vi "virtualOSA_model_code.vi"(11 "virtual OSA model":T1) -> (1 "OSA series":enum16{"OSA200", "OSA300", "UNKNOWN"}(ring), 3 "virtualOSA code":u16)   [LabVIEW 2010, in "OSA.lvclass"]
uses:
  OSA.lvclass
  _misc/Thorlabs_FTS_misc.llb/OSA_virtualModel.ctl
  OSA20X_misc.lvlib
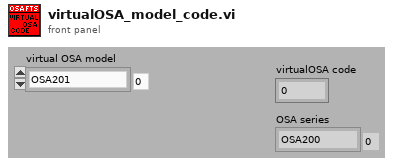
[diagram p1: front panel]
types:
  T1 = typedef "OSA20X_misc.lvlib/OSA_virtualModel.ctl" = enum16{"OSA201", "OSA201C", "OSA202", "OSA202C", "OSA203", "OSA203B", "OSA203C", "OSA205", "OSA205C", "REDSTONE301", "REDSTONE305"}
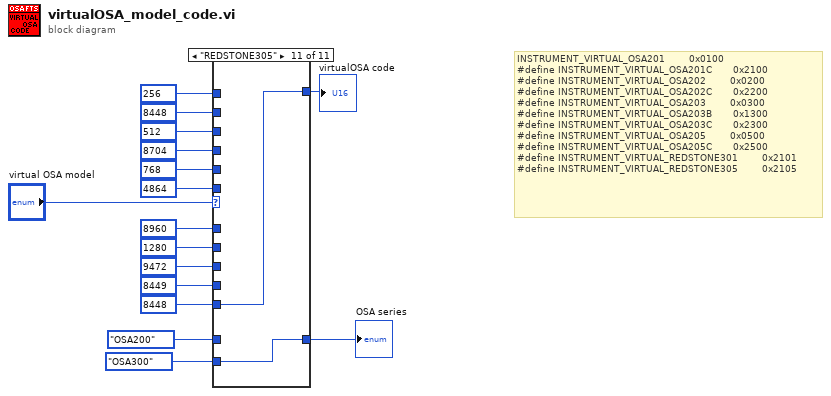
[diagram p0: block diagram]
diagram:
  # "INSTRUMENT_VIRTUAL_OSA201        0x0100\n#define INSTRUMENT_VIRTUAL_OSA201C       0x2100\n#define INSTRUMENT_VIRTUAL_OSA202        0x0200\n#define INSTRUMENT_VIRTUAL_OSA202C       0x2200\n#define INSTRUMENT_VIRTUAL_OSA203        0x0300\n#define INSTRUMENT_VIRTUAL_OSA203B       0x1300\n#define INSTRUMENT_VIRTUAL_OSA203C       0x2300\n#define INSTRUMENT_VIRTUAL_OSA205        0x0500\n#define INSTRUMENT_VIRTUAL_OSA205C       0x2500\n#define INSTRUMENT_VIRTUAL_REDSTONE301        0x2101\n#define INSTRUMENT_VIRTUAL_REDSTONE305        0x2105"
  n1 = case shown="\"REDSTONE305\"" "virtual OSA model" {
    tunnel: [w18 w20 w22 w24 w26 w28 w30 w32 w34 w36 w38] -> w4
    tunnel: u16 256 -> [w18 _ _ _ _ _ _ _ _ _ _]
    tunnel: u16 8448 -> [_ w20 _ _ _ _ _ _ _ _ _]
    tunnel: u16 512 -> [_ _ w22 _ _ _ _ _ _ _ _]
    tunnel: u16 8704 -> [_ _ _ w24 _ _ _ _ _ _ _]
    tunnel: u16 768 -> [_ _ _ _ w26 _ _ _ _ _ _]
    tunnel: u16 4864 -> [_ _ _ _ _ w28 _ _ _ _ _]
    tunnel: u16 8960 -> [_ _ _ _ _ _ w30 _ _ _ _]
    tunnel: u16 1280 -> [_ _ _ _ _ _ _ w32 _ _ _]
    tunnel: u16 9472 -> [_ _ _ _ _ _ _ _ w34 _ _]
    tunnel: u16 8449 -> [_ _ _ _ _ _ _ _ _ w36 _]
    tunnel: u16 8448 -> [_ _ _ _ _ _ _ _ _ _ w38]
    tunnel: enum16{"OSA200", "OSA300", "UNKNOWN"}."OSA200" ("OSA series") -> [w17 w19 w21 w23 w25 w27 w29 w31 w33 _ _]
    tunnel: [w17 w19 w21 w23 w25 w27 w29 w31 w33 w35 w37] -> w2
    tunnel: enum16{"OSA200", "OSA300", "UNKNOWN"}."OSA300" ("OSA series") -> [_ _ _ _ _ _ _ _ _ w35 w37]
    frame "OSA201", Default {
    }
    frame "OSA201C" {
    }
    frame "OSA202" {
    }
    frame "OSA202C" {
    }
    frame "OSA203" {
    }
    frame "OSA203B" {
    }
    frame "OSA203C" {
    }
    frame "OSA205" {
    }
    frame "OSA205C" {
    }
    frame "REDSTONE301" {
    }
    frame "REDSTONE305" {
    }
  }
  "virtualOSA code" <- w4
  "OSA series" <- w2
